vi "Emballage_BDD_supprime_case_vide_tableau.vi"(11 "Tableau IN":string[](array[string])) -> (3 "Tableau OUT":string[](array[string]))   [LabVIEW 2020]
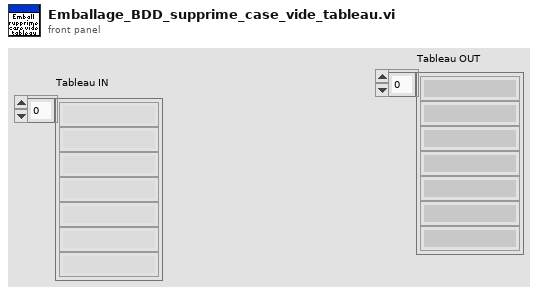
[diagram p1: front panel]
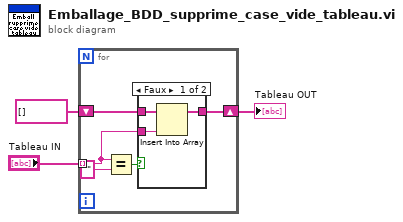
[diagram p0: block diagram]
diagram:
  n1 = for {
    tunnel: "Tableau IN" -> [w6] mode=indexing
    shift-right: [w7] -> w1
    shift-left: string[] [] -> [w8]
    n2 = Equal?(x=w6, y="") -> (x = y?=w4:bool)
    n3 = case shown="Faux" w4 {
      tunnel: w8 -> [w11 w12]
      tunnel: [w10 w12] -> w7
      tunnel: w6 -> [w9 _]
      frame False {
        n4 = Insert Into Array(array=w11, new element=w9) -> (w10:string[])  [unwired: 1 in]
      }
      frame True {
      }
    }
  }
  "Tableau OUT" <- w1
